vi "Get Line Name.vi"(8 "error in":errorcluster, 11 "Line":T1) -> (0 "error out":errorcluster, 2 "Name":string, 3 "Line 2":T1)   [LabVIEW 2013, in "Modbus Module configuration.lvclass"]
uses:
  Modbus Module configuration.lvclass
  Line.ctl
  module channel/Modbus Module Channel.lvclass
  <vilib>/NI/Tag Bus/tag/tag descriptor.lvclass/tag descriptor.ctl
  <vilib>/NI/Tag Bus/tag/tag descriptor.lvclass
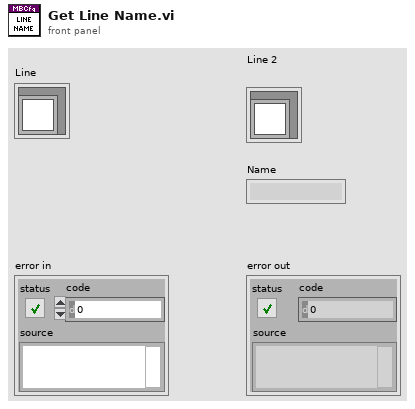
[diagram p1: front panel]
types:
  T1 = typedef "Modbus Module configuration.lvclass/Line.ctl" = cluster{"MB Channel":refnum<class "Modbus Module Channel.lvclass">}
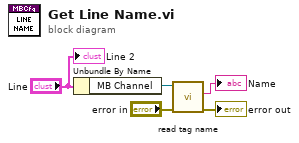
[diagram p0: block diagram]
diagram:
  n1 = Unbundle By Name("Line") -> ("MB Channel"=w5:refnum<class "Modbus Module Channel.lvclass">)
  n2 = call <vilib>:"read tag name.vi"("error in"="error in", "system tag in"=w5) -> ("error out"=→"error out":errorcluster, "name"=→"Name":string)  [unwired: 7 in, 1 out]
  "Line 2" <- "Line"
